vi "Message Log Mouse Down EHLC.vi"(8 "error in (no error)":errorcluster, 9 "Coords":T1, 10 "CtlRef":refnum<vi>, 11 "Message Log in":refnum<class "Message Log.lvclass">) -> (0 "error out":errorcluster, 3 "Message Log out":refnum<class "Message Log.lvclass">)   [LabVIEW 2017, in "Message Log.lvclass"]
uses:
  Message Log.lvclass
  <vilib>/Utility/miscctls.llb/LVPoint32TypeDef.ctl
  Listbox Selection.ctl
  <vilib>/Utility/miscctls.llb/LVRowAndColumnTypeDef.ctl
  rql_EHL Message Log - Mouse Down.ctl
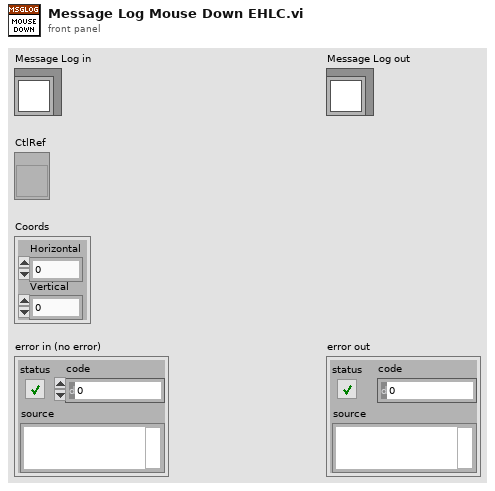
[diagram p1: front panel]
types:
  T1 = typedef "LVPoint32TypeDef.ctl" = cluster{"Horizontal":i32, "Vertical":i32}
  T2 = typedef "Message Log.lvclass/rql_EHL Message Log - Mouse Down.ctl" = cluster{"Listbox Selection":T3}
  T3 = typedef "Message Log.lvclass/Listbox Selection.ctl" = cluster{"Cell Position":T4, "Row":string[]}
  T4 = typedef "LVRowAndColumnTypeDef.ctl" = cluster{"Row":i32, "Column":i32}
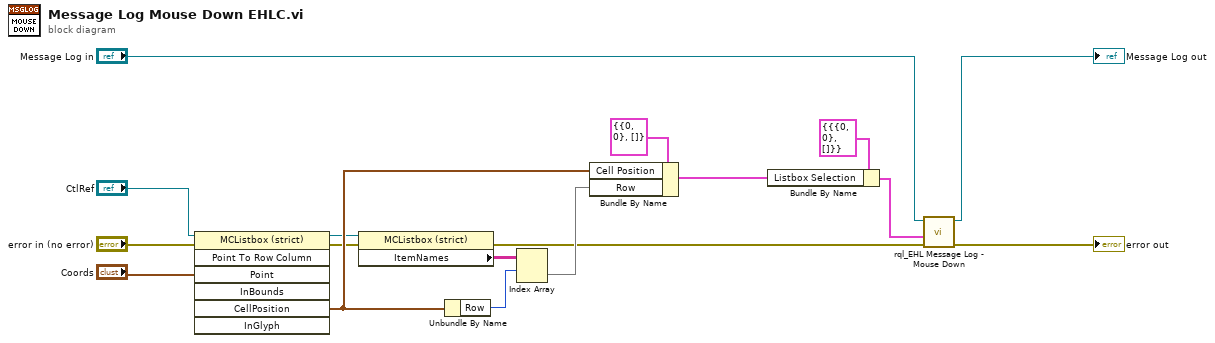
[diagram p0: block diagram]
diagram:
  n1 = invoke class="MCListbox (strict)" method="Point To Row Column"(reference="CtlRef", error in="error in (no error)", "Point"="Coords") -> (reference out=w15:refnum<vi>, error out=w12:errorcluster, "CellPosition"=w16:T4)  [unwired: 4 in, 4 out]
  n2 = property class="MCListbox (strict)"(reference=w15, error in=w12) -> (error out=w5:errorcluster, "ItemNames"=w13:string[][])  [unwired: 1 out]
  n3 = Unbundle By Name(w16) -> ("Row"=w14:i32)
  n4 = Index Array(array=w13, index (row)=w14) -> (element=w9:string[])  [unwired: 1 in]
  n5 = Bundle By Name(cluster=T3 {"Cell Position"={"Row"=0, "Column"=0}, "Row"=[]} ("Listbox Selection"), "Cell Position"=w16, "Row"=w9) -> (w3:T3)
  n6 = Bundle By Name(cluster=T2 {"Listbox Selection"={"Cell Position"={"Row"=0, "Column"=0}, "Row"=[]}} ("Data"), "Listbox Selection"=w3) -> (w1:T2)
  n7 = call "rql_EHL Message Log - Mouse Down.vi"("error in"=w5, "Data in"=w1, "Message Log in"="Message Log in") -> ("error out"=→"error out":errorcluster, "dup Message Log out"=→"Message Log out":refnum<class "Message Log.lvclass">)  [unwired: 7 in]
